vi "Lens Calibration.vi"(4 "Error In":errorcluster, 5 "File Path":path, 6 "Image In":T1) -> (0 "error out":errorcluster, 3 "Image Out":T1(plugin-control))   [LabVIEW 2017]
doc: "This VI will adjust for lens distortion in an image using a calibration file."
uses:
  <vilib>/vision/Image Controls.llb/IMAQ Image.ctl
  <vilib>/vision/NI_Vision_Development_Module.lvlib
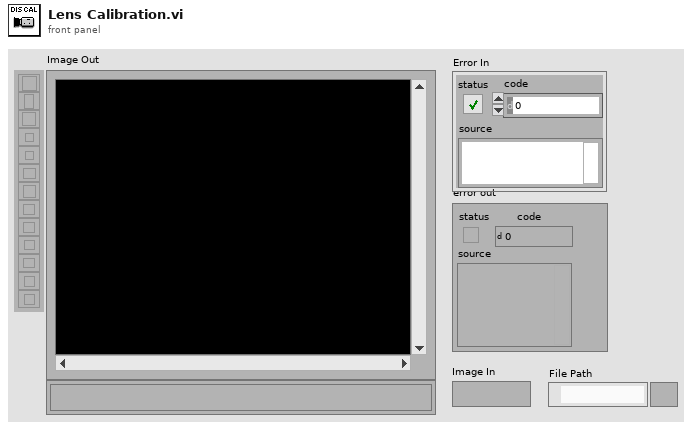
[diagram p1: front panel]
types:
  T1 = typedef "IMAQ Image.ctl" = refnum<image>
  T2 = cluster{"Origin Pixel":cluster{"X":sgl, "Y":sgl}, "Angle Relative to Horizontal (deg)":sgl, "Axis Reference":u32}
  T3 = cluster{"Origin Pixel":cluster{"X":sgl, "Y":sgl}, sgl, "Axis Reference":u32}
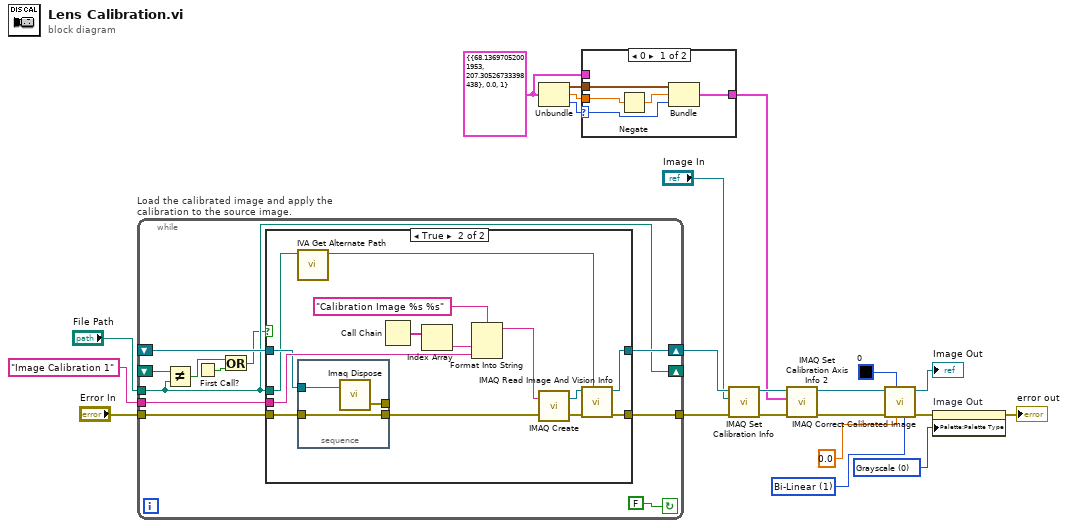
[diagram p0: block diagram]
diagram:
  w3 = u32 0 items=["Grayscale", "Binary", "Gradient", "Rainbow", "Temperature", "User Defined", "Binary 16 Bit", "Gradient 16 Bit", "Rainbow 16 Bit", "Temperature 16 Bit", "User Defined 16 Bit"] ("Palette Type")
  w11 = u32 1 items=["Zero Order", "Bi-Linear", "Quadratic", "Cubic Spline"] ("Interpolation Type")
  w15 = T2 {"Origin Pixel"={"X"=68.13697, "Y"=207.30527}, "Angle Relative to Horizontal (deg)"=0.0, "Axis Reference"=1} ("Calibration Axis Info")
  n1 = while "Load the calibrated image and apply the calibration to the source image." {
    shift-right: [w33] -> w22
    shift-left: _ -> [w32]
    tunnel: [w30] -> w21
    tunnel: "Error In" -> [w29]
    tunnel: "File Path" -> [w26]
    tunnel: "Image Calibration 1" ("Step Name") -> [w28]
    shift-right: [w26] -> _
    shift-left: _ -> [w27]
    stop <- FALSE continue-if-true
    n2 = Not Equal?(x=w27, y=w26) -> (x != y?=w24:bool)
    n3 = First Call?() -> (First Call?: T/F=w25:bool)
    n4 = Or(x=w24, y=w25) -> (x .or. y?=w23:bool)
    n5 = case shown="True" w23 {
      tunnel: [w35 w47] -> w33
      tunnel: w32 -> [w35 w39]
      tunnel: [w34 w44] -> w30
      tunnel: w29 -> [w34 w40]
      tunnel: w26 -> [_ w37]
      tunnel: w28 -> [_ w41]
      frame False {
      }
      frame True {
        n6 = call <vilib>:"IVA Get Alternate Path.vi"("Path In"=w37) -> ("Path Out"=w36:path)  [unwired: 10 out]
        n7 = stacked-sequence {
          tunnel: w40 -> [w51]
          tunnel: w39 -> [w52]
          tunnel: [w51] -> w38
          tunnel: [w50] -> _
          frame #0 {
            n8 = call "Imaq Dispose"("Image"=w52) -> ("error out"=w50:errorcluster)  [unwired: 2 in, 3 out]
          }
        }
        n9 = Call Chain() -> (call chain=w43:string[])
        n10 = Index Array(array=w43) -> (element=w42:string)  [unwired: 1 in]
        n11 = Format Into String(format string="Calibration Image %s %s" ("Image Name"), w42, w41) -> (resulting string=w49:string)  [unwired: 2 in, 1 out]
        n12 = call "IMAQ Create"("Image Name"=w49, "error in (no error)"=w38) -> ("New Image"=w46:T1, "error out"=w45:errorcluster)  [unwired: 2 in, 1 out]
        n13 = call "IMAQ Read Image And Vision Info"("File Path"=w36, "error in (no error)"=w45, "Image"=w46) -> ("error out"=w44:errorcluster, "Image Out"=w47:T1)  [unwired: 1 in, 6 out]
      }
    }
  }
  n14 = Unbundle(w15) -> ("Origin Pixel"=w12:cluster{"X":sgl, "Y":sgl}, "Angle Relative to Horizontal (deg)"=w13:sgl, "Axis Reference"=w16:u32)
  n15 = case shown="0" w16 {
    selector: w16 -> [w54 _]
    tunnel: w15 -> [_ w58]
    tunnel: [w53 w58] -> w14
    tunnel: w13 -> [w57 _]
    tunnel: w12 -> [w56 _]
    frame 0 {
      n16 = Negate(x=w57) -> (-x=w55:sgl)
      n17 = Bundle("Origin Pixel"=w56, w55, "Axis Reference"=w54) -> (w53:T3)  [unwired: 1 in]
    }
    frame 1, Default {
    }
  }
  n18 = call "IMAQ Set Calibration Info"("error in (no error)"=w21, "Image Dst"="Image In", "Image Src"=w22) -> ("error out"=w20:errorcluster, "Calibrated Image"=w17:T1)  [unwired: 1 in, 6 out]
  n19 = call-poly "IMAQ Set Calibration Axis Info 2"("error in (no error)"=w20, "Calibration Axis Info"=w14, "Calibration Template Image In"=w17) -> ("error out"=w18:errorcluster, "Calibration Template Image Out"=w10:T1)  [unwired: 7 out]
  n20 = call "IMAQ Correct Calibrated Image"("Interpolation Type"=w11, "Replace Value"=sgl 0.0, "Color Replace Value"=u32 0, "error in (no error)"=w18, "Image Src"=w10) -> ("error out"=w2:errorcluster, "Corrected Image"=→"Image Out":T1)  [unwired: 2 in, 3 out]
  n21 = property on="Image Out" class="ImageControl"(error in=w2, "Palette:Palette Type"=w3) -> (error out=→"error out":errorcluster)  [unwired: 1 in, 1 out]
